vi "build_DO_task.vi"(8 "error in":errorcluster) -> (0 "error out":errorcluster, 3 "task out":refnum<k21>)   [LabVIEW 2013]
uses:
  <vilib>/DAQmx/create/channels.llb/DAQmx Create Channel (DO-Digital Output).vi
  <resource>/objmgr/daqmx.rc
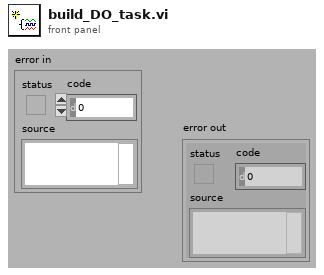
[diagram p1: front panel]
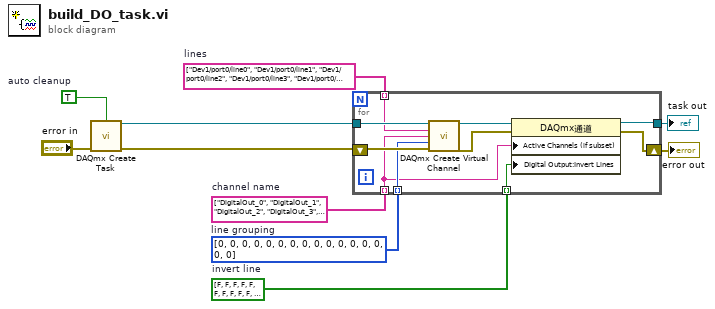
[diagram p0: block diagram]
diagram:
  w6 = bool[] [FALSE, FALSE, FALSE, FALSE, FALSE, FALSE, FALSE, FALSE, FALSE, FALSE, FALSE, FALSE, FALSE, FALSE, FALSE, FALSE]  # invert line
  w5 = i32[] [0, 0, 0, 0, 0, 0, 0, 0, 0, 0, 0, 0, 0, 0, 0, 0] items=["one channel for each line", "one channel for all lines"]  # line grouping
  w4 = string[] ["DigitalOut_0", "DigitalOut_1", "DigitalOut_2", "DigitalOut_3", "DigitalOut_4", "DigitalOut_5", "DigitalOut_6", "DigitalOut_7", "DigitalOut_8", "DigitalOut_9", "DigitalOut_10", "DigitalOut_11", "DigitalOut_12", "DigitalOut_13", "DigitalOut_14", "DigitalOut_15"]  # channel name
  w3 = string[] ["Dev1/port0/line0", "Dev1/port0/line1", "Dev1/port0/line2", "Dev1/port0/line3", "Dev1/port0/line4", "Dev1/port0/line5", "Dev1/port0/line6", "Dev1/port0/line7", "Dev1/port0/line8", "Dev1/port0/line9", "Dev1/port0/line10", "Dev1/port0/line11", "Dev1/port0/line12", "Dev1/port0/line13", "Dev1/port0/line14", "Dev1/port0/line15"]  # lines
  w8 = TRUE  # auto cleanup
  n1 = call <vilib>:"DAQmx Create Task.vi"("auto cleanup"=w8, "error in"="error in") -> ("task out"=w7:refnum<k21>, "error out"=w9:errorcluster)  [unwired: 12 in]
  n2 = for {
    tunnel: w7 -> [w20]
    tunnel: w6 -> [w14] mode=indexing
    tunnel: w5 -> [w17] mode=indexing
    tunnel: w4 -> [w13] mode=indexing
    tunnel: w3 -> [w18] mode=indexing
    tunnel: [w15] -> w2
    shift-right: [w11] -> w1
    shift-left: w9 -> [w19]
    n3 = call-poly <vilib>:"DAQmx Create Virtual Channel.vi"("task in"=w20, "lines"=w18, "name to assign"=w13, "line grouping"=w17, "error in"=w19) -> ("task out"=w16:refnum<k21>, "error out"=w12:errorcluster)  [unwired: 9 in]
    n4 = property class="DAQmx通道"(reference=w16, error in=w12, "Active Channels (if subset)"=w13, "Digital Output:Invert Lines"=w14) -> (reference out=w15:refnum<k21>, error out=w11:errorcluster)
  }
  "error out" <- w1
  "task out" <- w2
